vi "Init_Init.vi"(11 "Object":T1) -> ()   [LabVIEW 2020, in "FlexWorker_Provider.lvlib"]
uses:
  FlexWorker_Provider.lvlib
  <resource>/Framework/Providers/API/mxLvOverlayState.ctl
  <resource>/Framework/Providers/API/mxLvUpdateUI.ctl
  <resource>/Framework/Providers/API/ItemRef.ctl
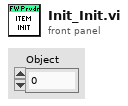
[diagram p1: front panel]
types:
  T1 = typedef "ItemRef.ctl" = u64
  T2 = typedef "mxLvUpdateUI.ctl" = cluster{"Action":u32, "Optional param 1":string, "Optional param 2":i32, "Optional param 3":string}
  T3 = typedef "mxLvOverlayState.ctl" = cluster{"Overlay Alias":string, "Active":bool}
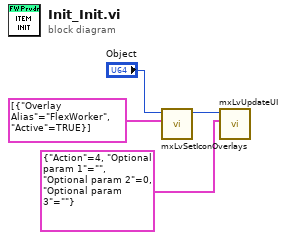
[diagram p0: block diagram]
diagram:
  n1 = call <resource>:"mxLvSetIconOverlays.vi"("Overlay States"=T3[] [{"Overlay Alias"="FlexWorker", "Active"=TRUE}], "Item"="Object") -> ("Item"=w2:T1)  [unwired: 8 in, 1 out]
  n2 = call <resource>:"mxLvUpdateUI.vi"("Update UI Settings"=T2 {"Action"=4, "Optional param 1"="", "Optional param 2"=0, "Optional param 3"=""}, "Item"=w2) -> ()  [unwired: 8 in, 2 out]
